vi "sub-import vi String.vi"(8 "error in (no error)":errorcluster caption="错误输入（无错误）", 11 "vi ref":refnum<vi>) -> (0 "error out":errorcluster caption="错误输出")   [LabVIEW 2011]
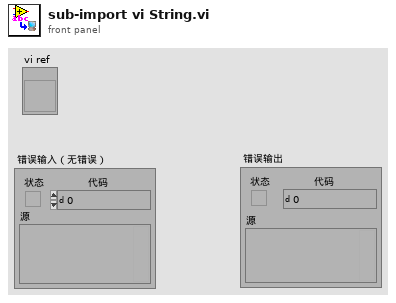
[diagram p1: front panel]
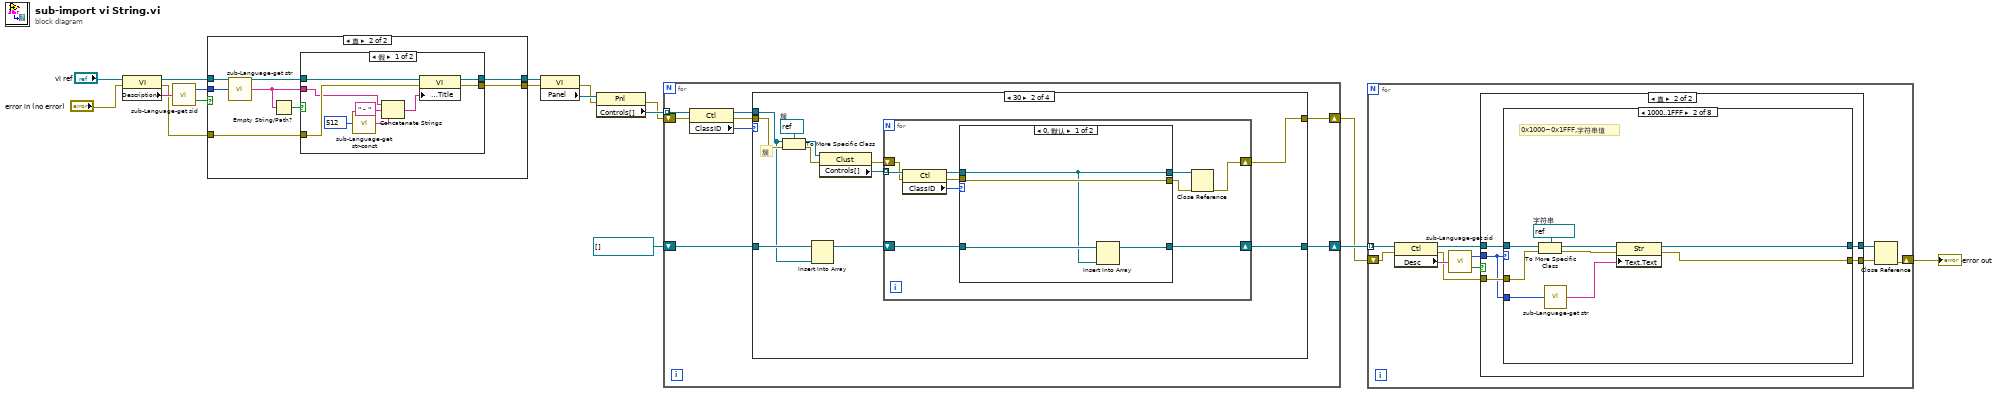
[diagram p0: block diagram]
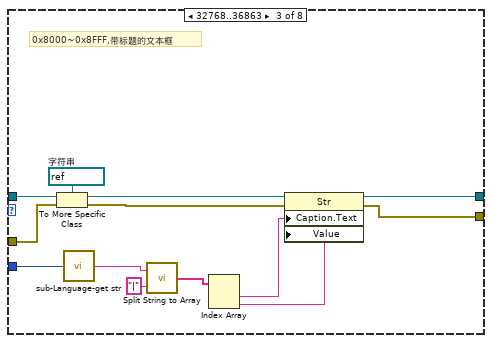
[diagram p4: hidden frame]
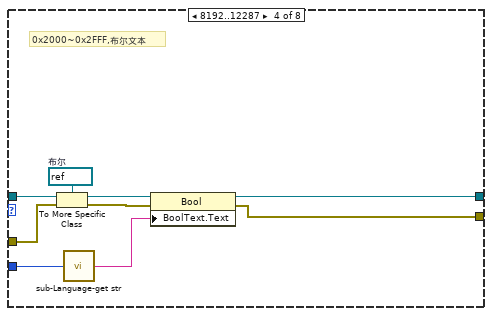
[diagram p5: hidden frame]
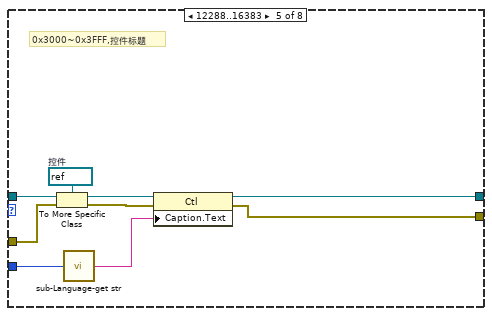
[diagram p6: hidden frame]
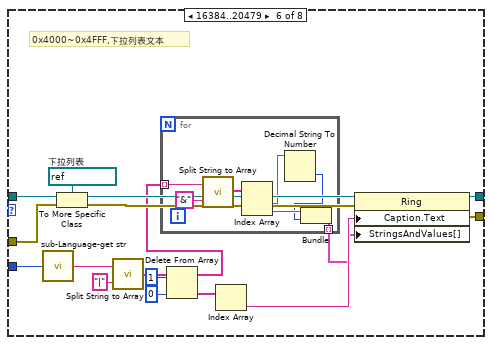
[diagram p7: hidden frame]
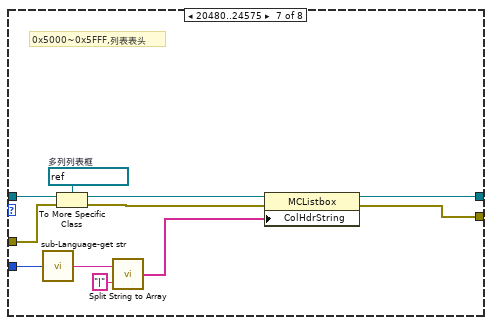
[diagram p8: hidden frame]
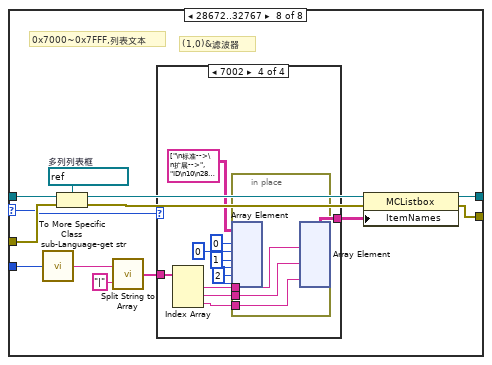
[diagram p9: hidden frame]
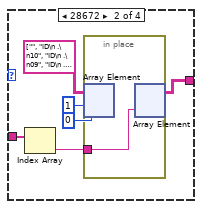
[diagram p11: hidden frame]
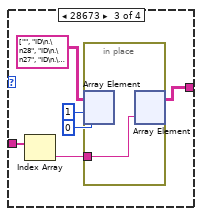
[diagram p12: hidden frame]
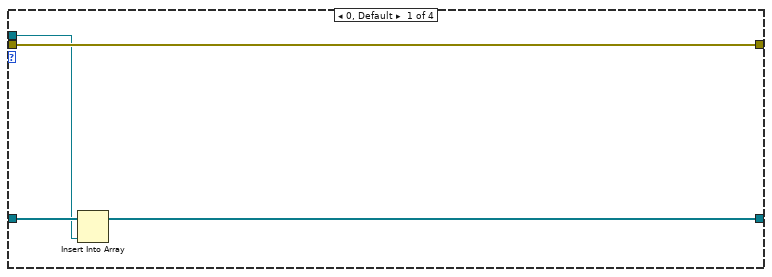
[diagram p13: hidden frame]
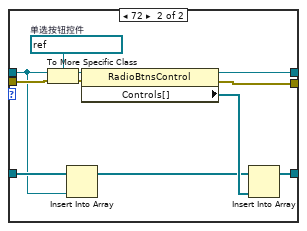
[diagram p14: hidden frame]
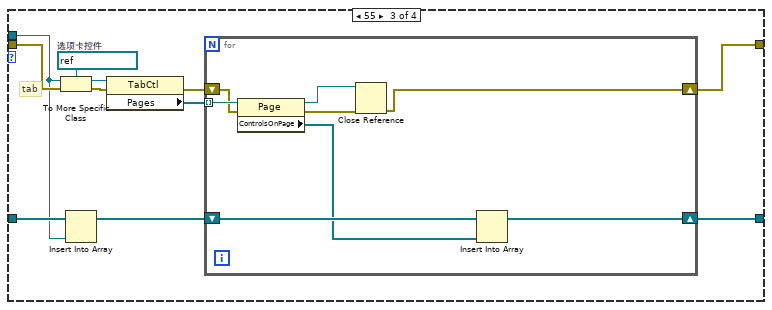
[diagram p15: hidden frame]
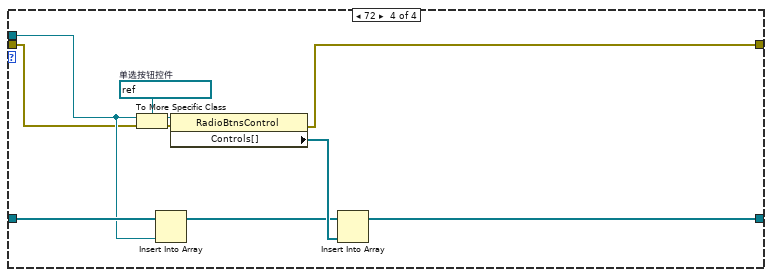
[diagram p16: hidden frame]
diagram:
  n1 = property class="VI"(reference="vi ref", error in="error in (no error)") -> (reference out=w12:refnum<vi>, error out=w11:errorcluster, "Description"=w15:string)
  n2 = call "sub-Language-get sid.vi"("str"=w15) -> ("sid"=w13:u32, "valid?"=w14:bool)
  n3 = case shown="真" w14 {
    tunnel: w13 -> [_ w26]
    tunnel: w12 -> [w19 w24]
    tunnel: w11 -> [w18 w22]
    tunnel: [w19 w21] -> w10
    tunnel: [w18 w20] -> w9
    frame False {
    }
    frame True {
      n4 = call-poly "sub-Language-get str.vi"("sid"=w26) -> ("str"=w23:string)
      n5 = Empty String/Path?(string/path=w23) -> (empty?=w25:bool)
      n6 = case shown="假" w25 {
        tunnel: w24 -> [w35 w37]
        tunnel: w23 -> [w30 _]
        tunnel: w22 -> [w34 w36]
        tunnel: [w33 w37] -> w21
        tunnel: [w32 w36] -> w20
        frame False {
          n7 = call "sub-Language-get str-const.vi"("sid"=u32 512) -> ("str"=w28:string)
          n8 = Concatenate Strings(w30, " - " ("字符串"), w28) -> (w27:string)
          n9 = property class="VI"(reference=w35, error in=w34, "Front Panel.Title"=w27) -> (reference out=w33:refnum<vi>, error out=w32:errorcluster)
        }
        frame True {
        }
      }
    }
  }
  n10 = property class="VI"(reference=w10, error in=w9) -> (error out=w7:errorcluster, "Panel"=w8:refnum<vi>)  [unwired: 1 out]
  n11 = property class="Pnl"(reference=w8, error in=w7) -> (error out=w5:errorcluster, "Controls[]"=w6:refnum<vi>[])  [unwired: 1 out]
  n12 = for {
    tunnel: w6 -> [w45] mode=indexing
    shift-right: [w40] -> w2
    shift-left: w5 -> [w44]
    shift-right: [w38] -> w3
    shift-left: refnum<vi>[] [] ("控件[]") -> [w39]
    n13 = property class="Ctl"(reference=w45, error in=w44) -> (reference out=w42:refnum<vi>, error out=w41:errorcluster, "ClassID"=w43:u32)
    n14 = case shown="30" w43 {
      tunnel: w42 -> [w47 w51 w91 w107]
      tunnel: w41 -> [w49 w60 w95 w106]
      tunnel: [w49 w54 w87 w105] -> w40
      tunnel: w39 -> [w48 w52 w92 w109]
      tunnel: [w46 w53 w86 w108] -> w38
      frame 0, Default {
        n15 = Insert Into Array(array=w48, new element=w47) -> (w46:refnum<vi>[])  [unwired: 1 in]
      }
      frame 30 {
        w59 = refnum<vi> refnum  # 簇
        # "簇"
        n16 = To More Specific Class(target class=w59, reference=w51, error in=w60) -> (specific class reference=w58:refnum<vi>, error out=w57:errorcluster)
        n17 = Insert Into Array(array=w52, new element=w51) -> (w50:refnum<vi>[])  [unwired: 1 in]
        n18 = property class="Clust"(reference=w58, error in=w57) -> (error out=w55:errorcluster, "Controls[]"=w56:refnum<vi>[])  [unwired: 1 out]
        n19 = for {
          tunnel: w56 -> [w70] mode=indexing
          shift-right: [w61] -> w54
          shift-left: w55 -> [w69]
          shift-right: [w64] -> w53
          shift-left: w50 -> [w65]
          n20 = property class="Ctl"(reference=w70, error in=w69) -> (reference out=w66:refnum<vi>, error out=w67:errorcluster, "ClassID"=w68:u32)
          n21 = case shown="0, 默认" w68 {
            tunnel: w67 -> [w74 w85]
            tunnel: w66 -> [w72 w76]
            tunnel: [w72 w81] -> w63
            tunnel: [w74 w80] -> w62
            tunnel: w65 -> [w73 w77]
            tunnel: [w71 w78] -> w64
            frame 0, Default {
              n22 = Insert Into Array(array=w73, new element=w72) -> (w71:refnum<vi>[])  [unwired: 1 in]
            }
            frame 72 {
              w84 = refnum<vi> refnum  # 单选按钮控件
              n23 = To More Specific Class(target class=w84, reference=w76, error in=w85) -> (specific class reference=w83:refnum<vi>, error out=w82:errorcluster)
              n24 = Insert Into Array(array=w77, new element=w76) -> (w75:refnum<vi>[])  [unwired: 1 in]
              n25 = property class="RadioBtnsControl"(reference=w83, error in=w82) -> (reference out=w81:refnum<vi>, error out=w80:errorcluster, "Controls[]"=w79:refnum<vi>[])
              n26 = Insert Into Array(array=w75, new element=w79) -> (w78:refnum<vi>[])  [unwired: 1 in]
            }
          }
          n27 = Close Reference(reference=w63, error in (no error)=w62) -> (error out=w61:errorcluster)
        }
      }
      frame 55 {
        w96 = refnum<vi> refnum  # 选项卡控件
        # "tab"
        n28 = To More Specific Class(target class=w96, reference=w91, error in=w95) -> (specific class reference=w93:refnum<vi>, error out=w94:errorcluster)
        n29 = Insert Into Array(array=w92, new element=w91) -> (w90:refnum<vi>[])  [unwired: 1 in]
        n30 = property class="TabCtl"(reference=w93, error in=w94) -> (error out=w88:errorcluster, "Pages"=w89:refnum<vi>[])  [unwired: 1 out]
        n31 = for {
          shift-right: [w98] -> w86
          shift-left: w90 -> [w99]
          tunnel: w89 -> [w104] mode=indexing
          shift-right: [w100] -> w87
          shift-left: w88 -> [w103]
          n32 = property class="Page"(reference=w104, error in=w103) -> (reference out=w102:refnum<vi>, error out=w101:errorcluster, "ControlsOnPage"=w97:refnum<vi>[])
          n33 = Close Reference(reference=w102, error in (no error)=w101) -> (error out=w100:errorcluster)
          n34 = Insert Into Array(array=w99, new element=w97) -> (w98:refnum<vi>[])  [unwired: 1 in]
        }
      }
      frame 72 {
        w114 = refnum<vi> refnum  # 单选按钮控件
        n35 = To More Specific Class(target class=w114, reference=w107, error in=w106) -> (specific class reference=w113:refnum<vi>, error out=w112:errorcluster)
        n36 = Insert Into Array(array=w109, new element=w107) -> (w110:refnum<vi>[])  [unwired: 1 in]
        n37 = property class="RadioBtnsControl"(reference=w113, error in=w112) -> (error out=w105:errorcluster, "Controls[]"=w111:refnum<vi>[])  [unwired: 1 out]
        n38 = Insert Into Array(array=w110, new element=w111) -> (w108:refnum<vi>[])  [unwired: 1 in]
      }
    }
  }
  n39 = for {
    tunnel: w3 -> [w124] mode=indexing
    shift-right: [w115] -> w1
    shift-left: w2 -> [w123]
    n40 = property class="Ctl"(reference=w124, error in=w123) -> (reference out=w119:refnum<vi>, error out=w118:errorcluster, "Desc"=w122:string)
    n41 = call "sub-Language-get sid.vi"("str"=w122) -> ("sid"=w120:u32, "valid?"=w121:bool)
    n42 = case shown="真" w121 {
      tunnel: w120 -> [_ w127]
      tunnel: w119 -> [w126 w131]
      tunnel: w118 -> [w125 w130]
      tunnel: [w126 w129] -> w116
      tunnel: [w125 w128] -> w117
      frame False {
      }
      frame True {
        n43 = case shown="1000..1FFF" w127 {
          selector: w127 -> [_ _ _ _ _ _ _ w211]
          tunnel: w131 -> [w133 w142 w155 w164 w173 w190 w208 w221]
          tunnel: w130 -> [w132 w141 w154 w163 w172 w189 w207 w220]
          tunnel: [w133 w137 w150 w159 w168 w185 w203 w216] -> w129
          tunnel: [w132 w136 w149 w158 w167 w184 w202 w215] -> w128
          tunnel: w127 -> [_ w135 w148 w157 w166 w183 w201 w214]
          frame 0..4095, Default {
            # "0x0000~0x0FFF,常量"
          }
          frame 4096..8191 {
            w140 = refnum<vi> refnum  # 字符串
            # "0x1000~0x1FFF,字符串值"
            n44 = To More Specific Class(target class=w140, reference=w142, error in=w141) -> (specific class reference=w139:refnum<vi>, error out=w138:errorcluster)
            n45 = call-poly "sub-Language-get str.vi"("sid"=w135) -> ("str"=w134:string)
            n46 = property class="Str"(reference=w139, error in=w138, "Text.Text"=w134) -> (reference out=w137:refnum<vi>, error out=w136:errorcluster)
          }
          frame 32768..36863 {
            w153 = refnum<vi> refnum  # 字符串
            # "0x8000~0x8FFF,带标题的文本框"
            n47 = To More Specific Class(target class=w153, reference=w155, error in=w154) -> (specific class reference=w152:refnum<vi>, error out=w151:errorcluster)
            n48 = call-poly "sub-Language-get str.vi"("sid"=w148) -> ("str"=w146:string)
            n49 = call "Split String to Array.vi"("搜索字符串/字符(-)"="|", "字符串"=w146) -> ("字符串数组"=w145:string[])
            n50 = Index Array(array=w145) -> (element #1=w144:string, element #2=w143:string)  [unwired: 2 in]
            n51 = property class="Str"(reference=w152, error in=w151, "Caption.Text"=w144, "Value"=w143) -> (reference out=w150:refnum<vi>, error out=w149:errorcluster)
          }
          frame 8192..12287 {
            w162 = refnum<vi> refnum  # 布尔
            # "0x2000~0x2FFF,布尔文本"
            n52 = To More Specific Class(target class=w162, reference=w164, error in=w163) -> (specific class reference=w161:refnum<vi>, error out=w160:errorcluster)
            n53 = call-poly "sub-Language-get str.vi"("sid"=w157) -> ("str"=w156:string)
            n54 = property class="Bool"(reference=w161, error in=w160, "BoolText.Text"=w156) -> (reference out=w159:refnum<vi>, error out=w158:errorcluster)
          }
          frame 12288..16383 {
            w171 = refnum<vi> refnum  # 控件
            # "0x3000~0x3FFF,控件标题"
            n55 = To More Specific Class(target class=w171, reference=w173, error in=w172) -> (specific class reference=w170:refnum<vi>, error out=w169:errorcluster)
            n56 = call-poly "sub-Language-get str.vi"("sid"=w166) -> ("str"=w165:string)
            n57 = property class="Ctl"(reference=w170, error in=w169, "Caption.Text"=w165) -> (reference out=w168:refnum<vi>, error out=w167:errorcluster)
          }
          frame 16384..20479 {
            w188 = refnum<vi> refnum  # 下拉列表
            # "0x4000~0x4FFF,下拉列表文本"
            n58 = call-poly "sub-Language-get str.vi"("sid"=w183) -> ("str"=w182:string)
            n59 = To More Specific Class(target class=w188, reference=w190, error in=w189) -> (specific class reference=w187:refnum<vi>, error out=w186:errorcluster)
            n60 = call "Split String to Array.vi"("搜索字符串/字符(-)"="|", "字符串"=w182) -> ("字符串数组"=w180:string[])
            n61 = Delete From Array(array=w180, length=1 ("长度"), index=0 ("索引")) -> (deleted portion=w177:string[], array with subset deleted=w175:string[])
            n62 = for {
              tunnel: w175 -> [w197] mode=indexing
              tunnel: [w191] -> w174 mode=indexing
              n63 = call "Split String to Array.vi"("搜索字符串/字符(-)"="&", "字符串"=w197) -> ("字符串数组"=w195:string[])
              n64 = Index Array(array=w195) -> (element #1=w194:string, element #2=w193:string)  [unwired: 2 in]
              n65 = Decimal String To Number(string=w194) -> (number=w192:i32)  [unwired: 2 in, 1 out]
              n66 = Bundle(w193, w192) -> (w191:cluster{string, i32})  [unwired: 1 in]
            }
            n67 = Index Array(array=w177) -> (element=w176:string)  [unwired: 1 in]
            n68 = property class="Ring"(reference=w187, error in=w186, "Caption.Text"=w176, "StringsAndValues[]"=w174) -> (reference out=w185:refnum<vi>, error out=w184:errorcluster)
          }
          frame 20480..24575 {
            w206 = refnum<vi> refnum  # 多列列表框
            # "0x5000~0x5FFF,列表表头"
            n69 = call-poly "sub-Language-get str.vi"("sid"=w201) -> ("str"=w200:string)
            n70 = To More Specific Class(target class=w206, reference=w208, error in=w207) -> (specific class reference=w205:refnum<vi>, error out=w204:errorcluster)
            n71 = call "Split String to Array.vi"("搜索字符串/字符(-)"="|", "字符串"=w200) -> ("字符串数组"=w198:string[])
            n72 = property class="MCListbox"(reference=w205, error in=w204, "ColHdrString"=w198) -> (reference out=w203:refnum<vi>, error out=w202:errorcluster)
          }
          frame 28672..32767 {
            w219 = refnum<vi> refnum  # 多列列表框
            # "(1,0)&滤波器"
            # "0x7000~0x7FFF,列表文本"
            n73 = call-poly "sub-Language-get str.vi"("sid"=w214) -> ("str"=w213:string)
            n74 = To More Specific Class(target class=w219, reference=w221, error in=w220) -> (specific class reference=w218:refnum<vi>, error out=w217:errorcluster)
            n75 = call "Split String to Array.vi"("搜索字符串/字符(-)"="|", "字符串"=w213) -> ("字符串数组"=w210:string[])
            n76 = case shown="7002" w211 {
              tunnel: w210 -> [_ w227 w234 w245]
              tunnel: [_ w224 w232 w243] -> w209
              frame 0, Default {
              }
              frame 28672 {
                n77 = Index Array(array=w227) -> (element=w225:string)  [unwired: 1 in]
                n78 = in-place {
                  in-place-border: w225 -> [w228]
                  n79 = in-place-array #1(string[][] [["", "ID\n .\n10", "ID\n .\n09", "ID\n .\n08", "", "ID\n .\n07", "ID\n .\n06", "ID\n .\n05", "ID\n .\n04", "ID\n .\n03", "ID\n .\n02", "ID\n .\n01", "ID\n .\n00"], ["滤波器\n\n", "\n", "", "", "", "", "", "", "", "", "", "", ""]] ("项名"), 1, 0) -> ()  [unwired: 1 out]
                  n80 = in-place-array #1(w228) -> (w224:string[][])  [unwired: 2 out]
                }
              }
              frame 28673 {
                n81 = Index Array(array=w234) -> (element=w233:string)  [unwired: 1 in]
                n82 = in-place {
                  in-place-border: w233 -> [w235]
                  n83 = in-place-array #2(string[][] [["", "ID\n.\n28", "ID\n.\n27", "ID\n.\n26", "ID\n.\n25", "ID\n.\n24", "", "ID\n.\n23", "ID\n.\n22", "ID\n.\n21", "ID\n.\n20", "ID\n.\n19", "ID\n.\n18", "ID\n.\n17", "ID\n.\n16", "", "ID\n.\n15", "ID\n.\n14", "ID\n.\n13", "ID\n.\n12", "ID\n.\n11", "ID\n.\n10", "ID\n.\n09", "ID\n.\n08", "", "ID\n.\n07", "ID\n.\n06", "ID\n.\n05", "ID\n.\n04", "ID\n.\n03", "ID\n.\n02", "ID\n.\n01", "ID\n.\n00"], ["滤波器\n\n", "\n", "", "", "", "", "", "", "", "", "", "", "", "", "", "", "", "", "", "", "", "", "", "", "", "", "", "", "", "", "", "", ""]] ("项名 2"), 1, 0) -> ()  [unwired: 1 out]
                  n84 = in-place-array #2(w235) -> (w232:string[][])  [unwired: 2 out]
                }
              }
              frame 28674 {
                w238 = 0
                n85 = Index Array(array=w245) -> (element #1=w244:string, element #2=w239:string, element #3=w236:string)  [unwired: 3 in]
                n86 = in-place {
                  in-place-border: w244 -> [w248]
                  in-place-border: w239 -> [w247]
                  in-place-border: w236 -> [w246]
                  n87 = in-place-array #3(string[][] [["\n标准-->\n扩展-->", "ID\n10\n28", "ID\n09\n27", "ID\n08\n26", "ID\n07\n25", "ID\n06\n24", "", "ID\n05\n23", "ID\n04\n22", "ID\n03\n21", "ID\n02\n20", "ID\n01\n19", "ID\n00\n18", "ID\n .\n17", "ID\n .\n16", "", "ID\n .\n15", "ID\n .\n14", "ID\n .\n13", "ID\n .\n12", "ID\n .\n11", "ID\n .\n10", "ID\n .\n09", "ID\n .\n08", "", "ID\n .\n07", "ID\n .\n06", "ID\n .\n05", "ID\n .\n04", "ID\n .\n03", "ID\n .\n02", "ID\n .\n01", "ID\n .\n00"], ["滤波器\n-扩展\n", "\n", "", "", "", "", "", "", "", "", "", "", "", "", "", "", "", "", "", "", "", "", "", "", "", "", "", "", "", "", "", "", ""], ["滤波器\n-标准\n", "", "", "", "", "", "", "", "", "", "", "", "", "", "", "", "", "", "", "", "", "", "", "", "", "", "", "", "", "", "", "", ""]] ("项名 3"), 0, w238, 1, w238, 2, w238) -> ()  [unwired: 3 out]
                  n88 = in-place-array #3(w248, w247, w246) -> (w243:string[][])  [unwired: 6 out]
                }
              }
            }
            n89 = property class="MCListbox"(reference=w218, error in=w217, "ItemNames"=w209) -> (reference out=w216:refnum<vi>, error out=w215:errorcluster)
          }
        }
      }
    }
    n90 = Close Reference(reference=w116, error in (no error)=w117) -> (error out=w115:errorcluster)
  }
  "error out" <- w1
